vi "Create AFDX IP (Source).vi"(11 "Source Info":T1={"domainID"=0, "sideID"=0, "locationID"=0, "partitionID"=1}) -> (3 "ip address":string)   [LabVIEW 2020, in "EthFrameManagement.lvlib"]
uses:
  EthFrameManagement.lvlib
  controls/ip_src_info_afdx.ctl
panel:
  out "network address":u32
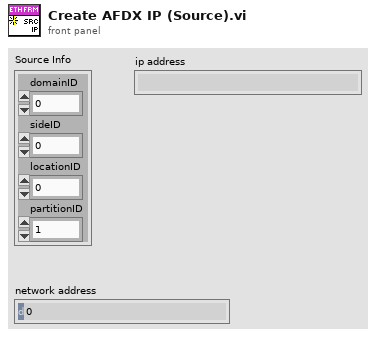
[diagram p1: front panel]
types:
  T1 = typedef "EthFrameManagement.lvlib/ip_src_info_afdx.ctl" = cluster{"domainID":u8, "sideID":u8, "locationID":u8, "partitionID":u8}
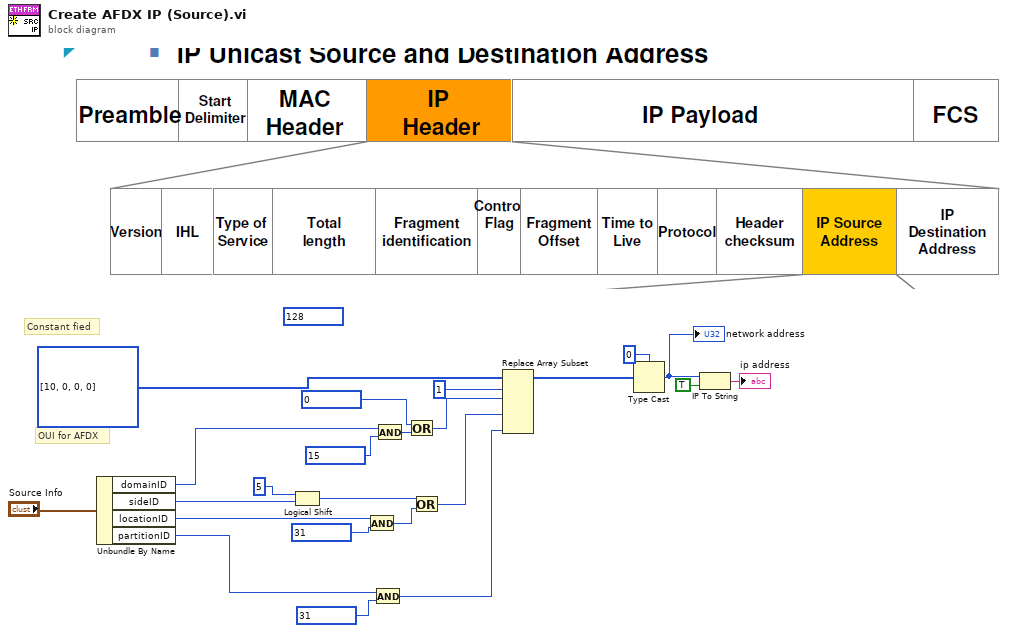
[diagram p0: block diagram]
diagram:
  (unwired) u8 128 ("y")
  # "OUI for AFDX"
  # "Constant fied"
  n1 = Unbundle By Name("Source Info") -> ("domainID"=w21:u8, "sideID"=w16:u8, "locationID"=w13:u8, "partitionID"=w17:u8)
  n2 = Logical Shift(y=i16 5, x=w16) -> (x << y=w12:u8)
  n3 = And(x=w13, y=u8 31) -> (x .and. y?=w11:u8)
  n4 = And(x=w17, y=u8 31) -> (x .and. y?=w9:u8)
  n5 = And(x=w21, y=u8 15) -> (x .and. y?=w3:u8)
  n6 = Or(x=u8 0 ("y"), y=w3) -> (x .or. y?=w2:u8)
  n7 = Or(x=w12, y=w11) -> (x .or. y?=w10:u8)
  n8 = Replace Array Subset(array=u8[] [10, 0, 0, 0] ("MAC-src"), new element #1=w2, index #1=1 ("index"), new element #2=w10, new element #3=w9) -> (w8:u8[])  [unwired: 2 in]
  n9 = Type Cast(type=u32 0, x=w8) -> (*(type *) &x=w6:u32)
  "network address" <- w6
  n10 = IP To String(1:TRUE ("dot notation? (F)"), 2:w6) -> (0:→"ip address":string)
